vi "Read-Save DefaultTemplate.vi"(6 "Task":enum16{"Save", "Read"}(ring), 11 "Template":string) -> (0 "Pref Path":path, 3 "Template Out":string)   [LabVIEW 2024]
uses:
  Mic/Mic_Global.vi
panel:
  out "text":string
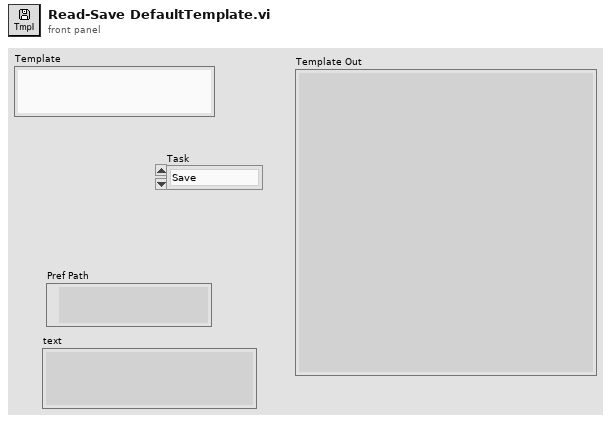
[diagram p1: front panel]
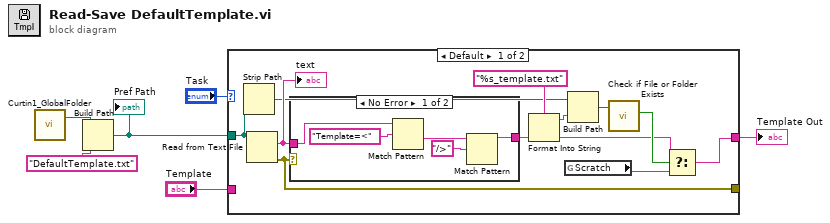
[diagram p0: block diagram]
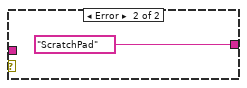
[diagram p2: hidden frame]
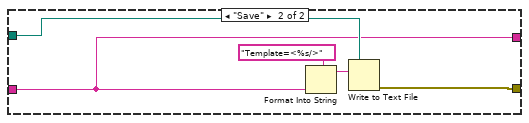
[diagram p3: hidden frame]
diagram:
  n1 = call "Curtin1_GlobalFolder.vi"() -> ("LabVIEW Data Path"=w1:path)  [unwired: 1 in, 1 out]
  n2 = Build Path(base path=w1, name or relative path="DefaultTemplate.txt") -> (appended path=w5:path)
  "Pref Path" <- w5
  n3 = case shown="Default" "Task" {
    tunnel: "Template" -> [_ w25]
    tunnel: w5 -> [w14 w28]
    tunnel: [w16 w26] -> _
    tunnel: [w9 w25] -> w2
    frame Default {
      n4 = Strip Path(path=w14) -> (stripped path=w7:path)  [unwired: 1 out]
      n5 = Read from Text File(file (use dialog)=w14) -> (text=w17:string, error out=w16:errorcluster)  [unwired: 3 in, 2 out]
      "text" <- w17
      n6 = case shown="No Error" w16 {
        tunnel: [w18 "ScratchPad" ("Notes")] -> w10
        tunnel: w17 -> [w22 _]
        frame No Error {
          n7 = Match Pattern(string=w22, regular expression="Template=<" ("format string")) -> (after substring=w21:string)  [unwired: 1 in, 3 out]
          n8 = Match Pattern(string=w21, regular expression="/>" ("format string")) -> (before substring=w18:string)  [unwired: 1 in, 3 out]
        }
        frame Error {
        }
      }
      n9 = Format Into String(format string="%s_template.txt", w10) -> (resulting string=w15:string)  [unwired: 2 in, 1 out]
      n10 = global read "Mic_Global.vi" "Scratch"() -> (w11:string)
      n11 = Build Path(base path=w7, name or relative path=w15) -> (appended path=w13:path)
      n12 = call <vilib>:"Check if File or Folder Exists.vi"("path"=w13) -> ("file or folder exists?"=w12:bool)  [unwired: 8 in, 2 out]
      n13 = Select(t=w10, s=w12, f=w11) -> (s? t:f=w9:string)
    }
    frame "Save" {
      n14 = Format Into String(format string="Template=<%s/>", w25) -> (resulting string=w27:string)  [unwired: 2 in, 1 out]
      n15 = Write to Text File(file (use dialog)=w28, text=w27) -> (error out=w26:errorcluster)  [unwired: 2 in, 2 out]
    }
  }
  "Template Out" <- w2
